vi "Find Handle by Ref.vi"(8 "error in (no error)":errorcluster, 10 "Ref":refnum<vi>, 11 "BetterHandle array":refnum<class "BetterHandle.lvclass">[](array[class])) -> (0 "error out":errorcluster, 2 "Handle index":i32, 3 "BetterHandle array":refnum<class "BetterHandle.lvclass">[](array[class]))   [LabVIEW 2020, in "BetterDragAndDrop.lvlib" / "BetterHandle.lvclass"]
uses:
  BetterHandle.lvclass
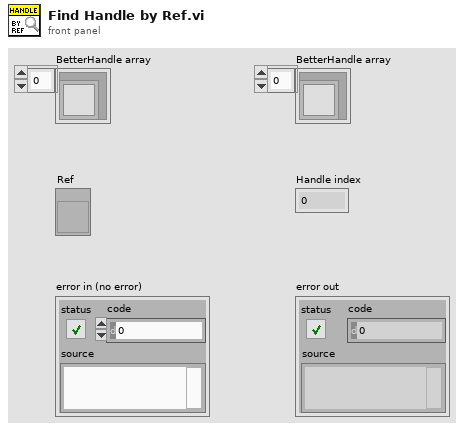
[diagram p1: front panel]
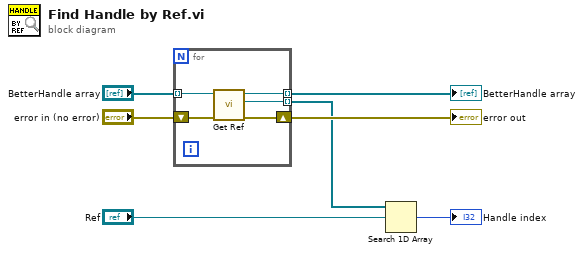
[diagram p0: block diagram]
diagram:
  n1 = for {
    tunnel: "BetterHandle array" -> [w12] mode=indexing
    tunnel: [w11] -> w6 mode=indexing
    tunnel: [w10] -> w2 mode=indexing
    shift-right: [w8] -> w4
    shift-left: "error in (no error)" -> [w9]
    n2 = call-dynamic "Get Ref.vi"("error in (no error)"=w9, "BetterHandle in"=w12) -> ("error out"=w8:errorcluster, "Tree/LB/MCL ref"=w10:refnum<vi>, "BetterHandle out"=w11:refnum<class "BetterHandle.lvclass">)  [unwired: 7 in]
  }
  "BetterHandle array" <- w6
  "error out" <- w4
  n3 = Search 1D Array(1D array=w2, element="Ref") -> (index of element=→"Handle index":i32)  [unwired: 1 in]
